vi "update_attrs.vi"(8 "error in (no error)":errorcluster, 10 "Nested Enqueuers Map":T1(c390), 11 "UDP_transmitter in":refnum<class "UDP_transmitter.lvclass">) -> (0 "error out":errorcluster, 3 "UDP_transmitter out":refnum<class "UDP_transmitter.lvclass">)   [LabVIEW 2025, in "UDP_transmitter.lvlib" / "UDP_transmitter.lvclass"]
uses:
  UDP_transmitter.lvclass
  <vilib>/ActorFramework/Message Enqueuer/Message Enqueuer.lvclass
  UDP_transmitter.lvclass/UDP_transmitter.ctl
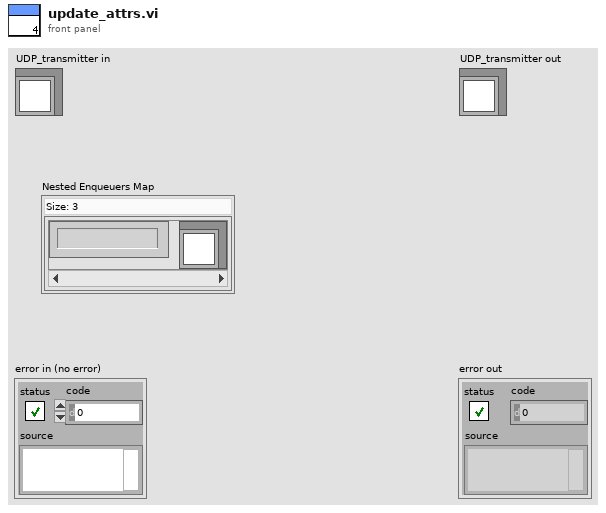
[diagram p1: front panel]
types:
  T1 = map{string, refnum<class "Message Enqueuer.lvclass">}
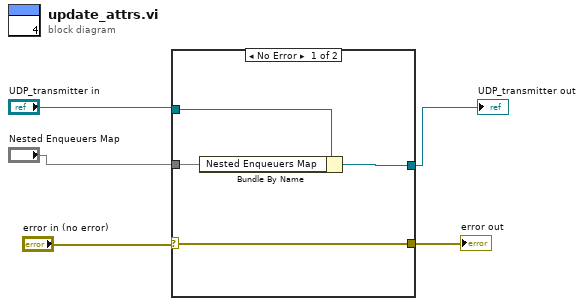
[diagram p0: block diagram]
diagram:
  n1 = case shown="No Error" "error in (no error)" {
    selector: "error in (no error)" -> [w6 w10]
    tunnel: "UDP_transmitter in" -> [w9 w11]
    tunnel: [w8 w11] -> w4
    tunnel: "Nested Enqueuers Map" -> [w7 _]
    tunnel: [w6 w10] -> w3
    frame No Error {
      n2 = Bundle By Name(cluster=w9, "Nested Enqueuers Map"=w7) -> (w8:refnum<class "UDP_transmitter.lvclass">)
    }
    frame Error {
    }
  }
  "error out" <- w3
  "UDP_transmitter out" <- w4
